vi "Drive Immediate.vi"(4 "Brake":bool, 6 "Shift":i32, 7 "Description":string, 8 "Command Info In":T1, 10 "Right Setpoint":dbl, 11 "Left Setpoint":dbl) -> (0 "Command Info Out":T1)   [LabVIEW 2016]
doc: "Often used for joystick control, this VI checks to see that the joystick axes are outside the deadband and updates the motors appropriately."
uses:
  <vilib>/Rock Robotics/WPI/Framework/Command Status Info.ctl
  <vilib>/Rock Robotics/WPI/Framework/Completion Status.ctl
  <vilib>/Rock Robotics/WPI/Framework/Completion Notifier.ctl
  Implementation/Drive Setpoints.ctl
  Implementation/Drive Operations.ctl
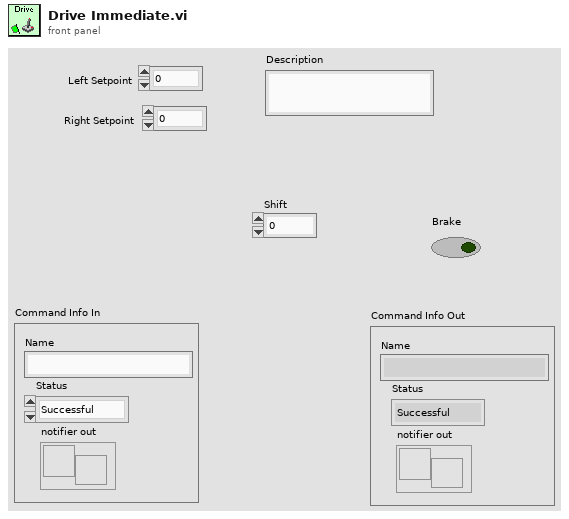
[diagram p1: front panel]
types:
  T1 = typedef "Command Status Info.ctl" = cluster{"Name":string, "Status":T2, "notifier out":T3}
  T2 = typedef "Completion Status.ctl" = enum16{"Successful", "Aborted", "Incomplete"}
  T3 = typedef "Completion Notifier.ctl" = refnum<notifier>
  T4 = typedef "Drive Setpoints.ctl" = cluster{"Operation":T5, "Left Setpoint":dbl, "Right Setpoint":dbl, "Duration":dbl, "Shift state":i8, "Angle":dbl, "Brake":bool}
  T5 = typedef "Drive Operations.ctl" = enum16{"Reserve", "Read Current", "Immediate", "Drive for Time", "Drive for Distance", "Turn to angle", "Vision Turn", "Vision close distance", "Reset Gyro", "Turn until target", "Brake", "One side PID drive straight", "DriveStraight"}
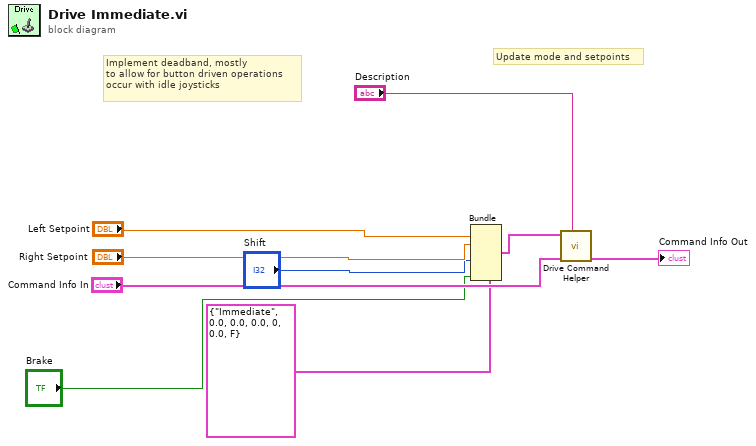
[diagram p0: block diagram]
diagram:
  # "Implement deadband, mostly\nto allow for button driven operations\noccur with idle joysticks"
  # "Update mode and setpoints"
  n1 = Bundle(cluster=T4 {"Operation"=enum."Immediate", "Left Setpoint"=0.0, "Right Setpoint"=0.0, "Duration"=0.0, "Shift state"=0, "Angle"=0.0, "Brake"=FALSE} ("SubSystem Data"), "Left Setpoint"="Left Setpoint", "Right Setpoint"="Right Setpoint", "Shift state"="Shift", "Brake"="Brake") -> (w1:T4)  [unwired: 3 in]
  n2 = call "Drive Command Helper.vi"("Description"="Description", "Command Info In"="Command Info In", "SubSystem Data"=w1) -> ("Command Info Out"=→"Command Info Out":T1)  [unwired: 7 in, 1 out]
